vi "Read From Queue.vi"(8 "error in (no error)":errorcluster, 11 "BehaviorData in":refnum<class "BehaviorData.lvclass">) -> (0 "error out":errorcluster, 2 "Array":waveform(dbl)[](array[waveform]), 3 "BehaviorData out":refnum<class "BehaviorData.lvclass">)   [LabVIEW 2011, in "BehaviorData.lvclass"]
uses:
  BehaviorData.lvclass
  BehaviorData.lvclass/BehaviorData.ctl
  <vilib>/Analysis/polynomials.llb/2D Polynomial Evaluation (DBL).vi
  <vilib>/Analysis/NI_AALPro.lvlib
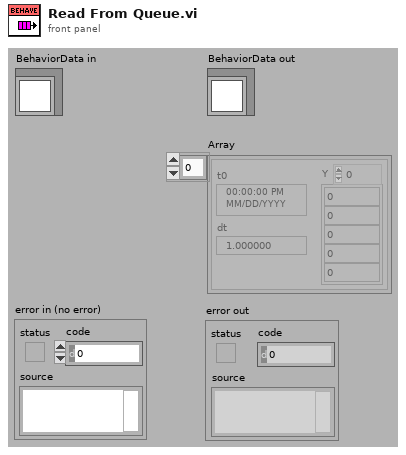
[diagram p1: front panel]
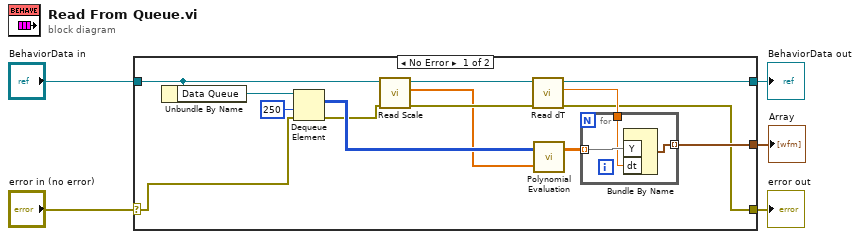
[diagram p0: block diagram]
diagram:
  n1 = case shown="No Error" "error in (no error)" {
    selector: "error in (no error)" -> [w18 w24]
    tunnel: [w13 w24] -> w4
    tunnel: [w14 w23] -> w2
    tunnel: "BehaviorData in" -> [w10 w23]
    tunnel: [w15 _] -> w1
    frame No Error {
      n2 = Unbundle By Name(w10) -> ("Data Queue"=w19:refnum<queue>)
      n3 = Dequeue Element(queue=w19, timeout in ms (-1)=250, error in (no error)=w18) -> (element=w12:i32[][], error out=w8:errorcluster)  [unwired: 2 out]
      n4 = call-dynamic "Read Scale.vi"("error in (no error)"=w8, "AcquireTraces in"=w10) -> ("error out"=w7:errorcluster, "Scale (V/LSB)"=w6:dbl[], "AcquireTraces out"=w9:refnum<class "BehaviorData.lvclass">)  [unwired: 7 in]
      n5 = call-dynamic "Read dT.vi"("error in (no error)"=w7, "AcquireTraces in"=w9) -> ("error out"=w13:errorcluster, "dT"=w16:dbl, "AcquireTraces out"=w14:refnum<class "BehaviorData.lvclass">)  [unwired: 7 in]
      n6 = call-poly <vilib>:"Polynomial Evaluation.vi"("P(x)"=w6, "A"=w12) -> ("P(A)"=w11:dbl[][])  [unwired: 1 out]
      n7 = for {
        tunnel: w11 -> [w22] mode=indexing
        tunnel: w16 -> [w21]
        tunnel: [w20] -> w15 mode=indexing
        n8 = Bundle By Name("Y"=w22, "dt"=w21) -> (w20:waveform(dbl))  [unwired: 1 in]
      }
    }
    frame Error {
    }
  }
  "error out" <- w4
  "BehaviorData out" <- w2
  "Array" <- w1
